vi "Write LV Version.vi"(8 "error in (no error)":errorcluster, 10 "LV Version":string="14.0", 11 "VIP Install in":refnum<class "VIPM Update.lvclass">) -> (0 "error out":errorcluster, 3 "VIP Install out":refnum<class "VIPM Update.lvclass">)   [LabVIEW 2014, in "VIPM Update.lvclass"]
uses:
  VIPM Update.lvclass
  VIPM Update.lvclass/VIPM Update.ctl
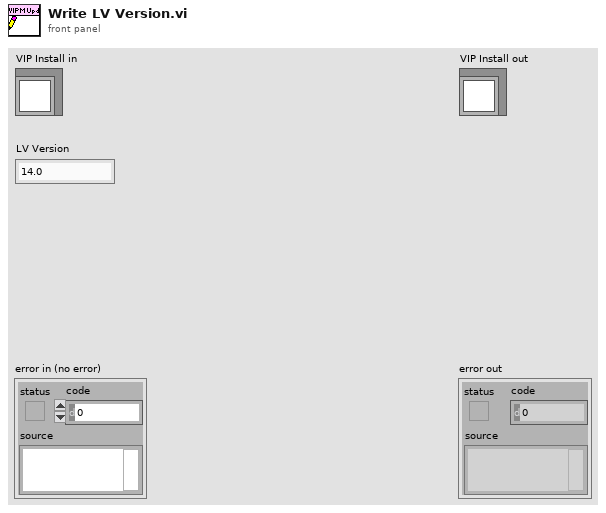
[diagram p1: front panel]
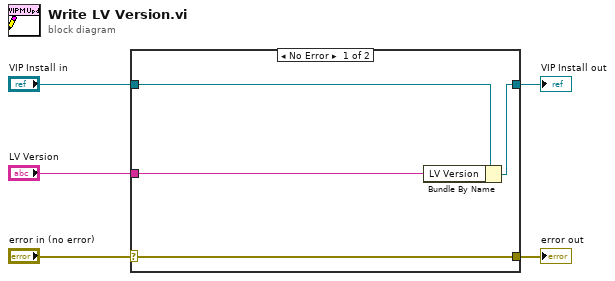
[diagram p0: block diagram]
diagram:
  n1 = case shown="No Error" "error in (no error)" {
    selector: "error in (no error)" -> [w9 w10]
    tunnel: [w9 w10] -> w4
    tunnel: [w7 w11] -> w2
    tunnel: "VIP Install in" -> [w8 w11]
    tunnel: "LV Version" -> [w6 _]
    frame No Error {
      n2 = Bundle By Name(cluster=w8, "LV Version"=w6) -> (w7:refnum<class "VIPM Update.lvclass">)
    }
    frame Error {
    }
  }
  "error out" <- w4
  "VIP Install out" <- w2
